vi "Comm_write 1d cdb.vi"(7 "Sample Offset":u64, 8 "error in (no error)":errorcluster, 9 "timeout in ms (0)":i32, 10 "Data":cdb[](array[numeric]), 11 "WPL Comm (1D CDB) in":refnum<class "WPL Comm (1D CDB).lvclass">) -> (0 "error out":errorcluster, 1 "timed out?":bool, 3 "WPL Comm (1D CDB) out":refnum<class "WPL Comm (1D CDB).lvclass">)   [LabVIEW 2020, in "Internal Comm Classes.lvlib" / "WPL Comm (1D CDB).lvclass"]
uses:
  WPL Comm (1D CDB).lvclass
  D:/p4/penguin/lvaddon/Veristand/master/src/LabVIEW/vilib/NI VeriStand/Custom Device Waveform API/Internal Comm Classes/WPL Comm/WPL Comm.lvclass
  WPL Comm (1D CDB).lvclass/WPL Comm (1D CDB).ctl
  WPL Command.ctl
  WPL Comm.lvclass/WPL Comm.ctl
  WPL Comm.lvclass
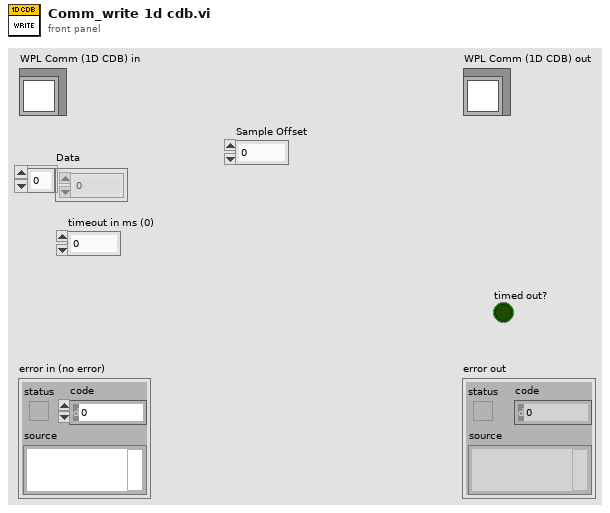
[diagram p1: front panel]
types:
  T1 = typedef "Internal Comm Classes.lvlib/WPL Comm (1D CDB).lvclass/Waveform 1d cdb queue.ctl" = refnum<queue>
  T2 = typedef "Internal Comm Classes.lvlib/WPL Comm.lvclass/WPL Command.ctl" = enum16{"Register 1D DBL Reader", "Unregister 1D DBL Reader", "Register 1D DBL Writer", "Register 2D DBL Writer", "Unregister 1D DBL Writer", "Unregister 2D DBL Writer", "DBL WFM Start", "WFM 1D DBL Data", "WFM 2D DBL Data", "Shut down", "Handle Error", "Register 1D CDB Reader", "Unregister 1D CDB Reader", "Register 1D CDB Writer", "Unregister 1D CDB Writer", "Register 2D CDB Writer", "Unregister 2D CDB Writer", "WFM 1D CDB Data", "WFM 2D CDB Data", "CDB WFM Start", "Error Shutdown", "Register Streams", "Unregister Streams", "Delete All Streams", "Get WFM DTs", "DBL WFM Multi Start", "CDB WFM Multi Start"}
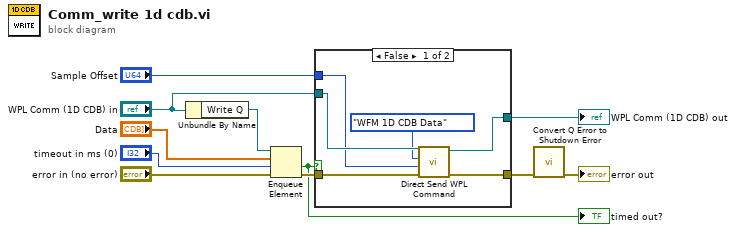
[diagram p0: block diagram]
diagram:
  n1 = Unbundle By Name("WPL Comm (1D CDB) in") -> ("Write Q"=w11:T1)
  n2 = Enqueue Element(queue=w11, element="Data", timeout in ms (-1)="timeout in ms (0)", error in (no error)="error in (no error)") -> (timed out?=w6:bool, error out=w7:errorcluster)  [unwired: 1 out]
  "timed out?" <- w6
  n3 = case shown="False" w6 {
    tunnel: w7 -> [w13 w19]
    tunnel: "Sample Offset" -> [w12 _]
    tunnel: "WPL Comm (1D CDB) in" -> [w17 w18]
    tunnel: [w14 w19] -> w2
    tunnel: [w15 w18] -> w3
    frame False {
      n4 = call "Direct Send WPL Command.vi"("error in (no error)"=w13, "SampleOffset"=w12, "Command"=WPL_Command."WFM 1D CDB Data", "WPL Comm"=w17) -> ("error out"=w14:errorcluster, "WPL Comm Dup"=w15:refnum<class "WPL Comm (1D CDB).lvclass">)  [unwired: 6 in]
    }
    frame True {
    }
  }
  "WPL Comm (1D CDB) out" <- w3
  n5 = call "Convert Q Error to Shutdown Error.vi"("error in (no error)"=w2) -> ("error out"=→"error out":errorcluster)  [unwired: 10 in]
